vi "test.vi"() -> ()   [LabVIEW 2013]
uses:
  lightfield-automation-labview/LightField Automation.lvclass
panel:
  in  "Delete File?":bool
  in  "Capture Frames":i32=-1
  in  "Capture":bool
  out "Capture ROI 1, Frame 1, Row 2":dbl[](graph)
  out "Acquire ROI 1, Frame 1, Row 1":dbl[](graph)
  in  "Acquire":bool
  in  "ExperimentName":string="Experiment4"
  out "Capture ROI 1, Frame 1":dbl[][](graph)
  out "Acquire ROI 1, Frame 1":dbl[][](graph)
  in  "?":bool
  out "Exposures Per Frame":i32=1
  in  "Exposures Per Frame":i32=1
  out "Number of Frames":i32=1
  in  "Number of Frames":i32=1
  out "Exposure Time (s)":dbl=0.10000000000000009
  in  "Exposure Time (s)":dbl=0.10000000000000009
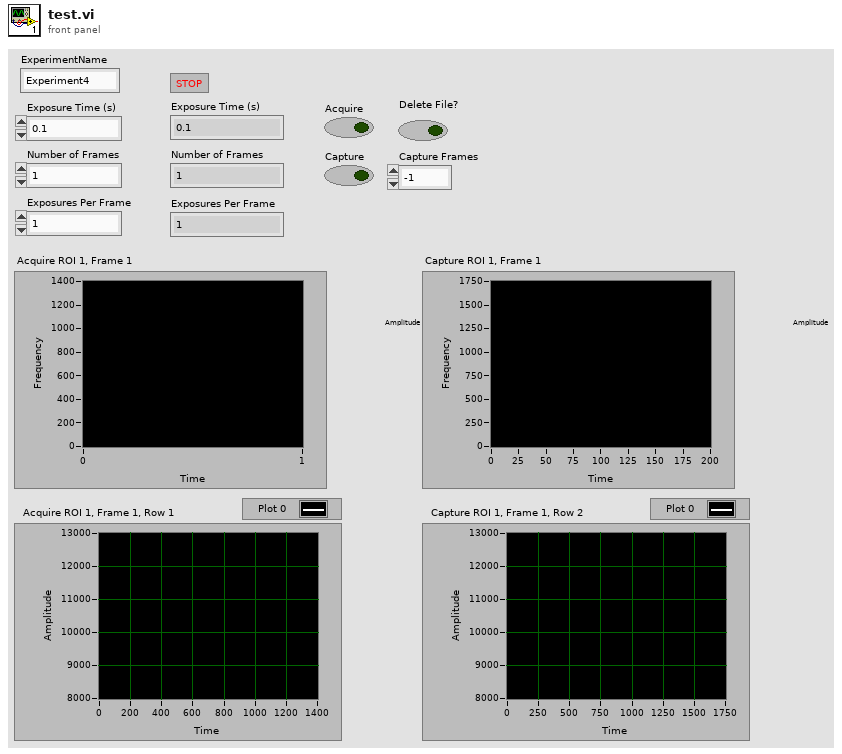
[diagram p1: front panel]
types:
  T1 = cluster{"Image":dbl[][][], "Frame Size":cluster{"F":i32, "Y":i32, "X":i32}}[]
  T2 = cluster{"Image":dbl[][][], "Frame Size":cluster{"F":i32, "Y":i32, "X":i32}}
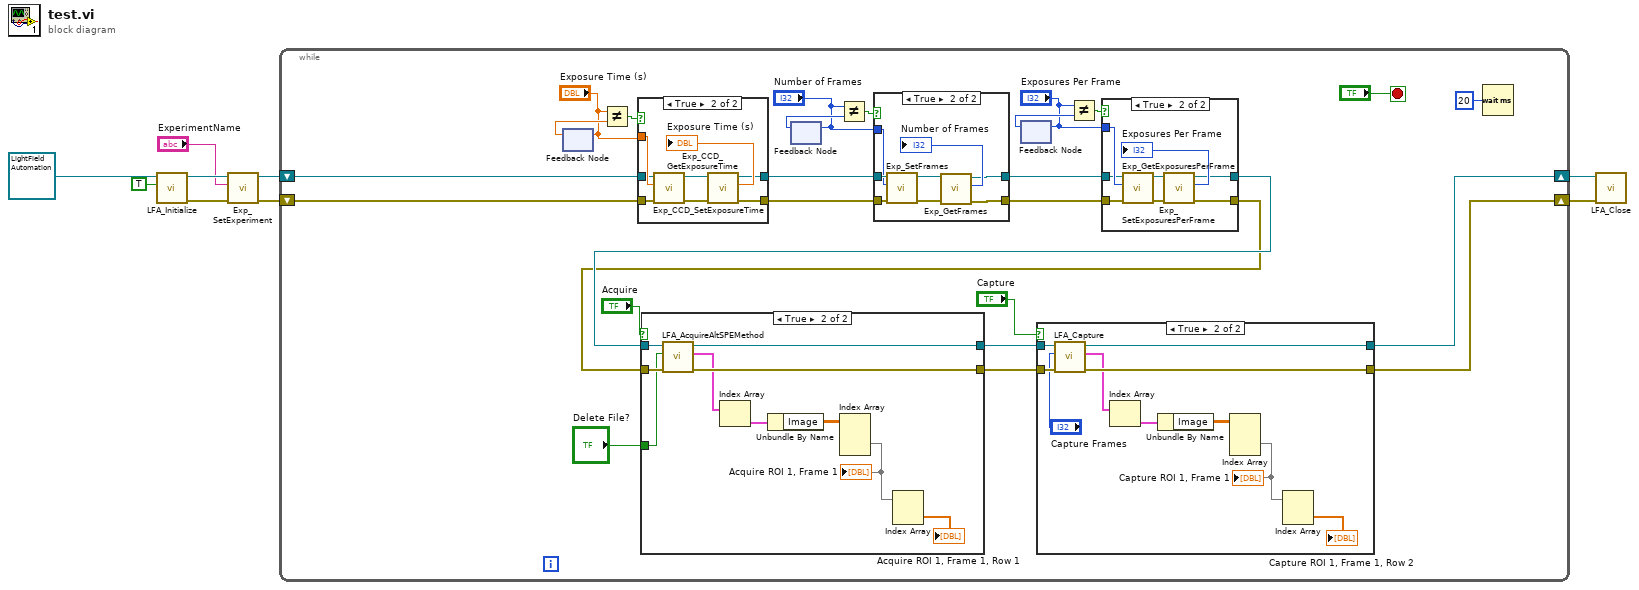
[diagram p0: block diagram]
diagram:
  n1 = call "LFA_Initialize.vi"("Is Visible?"=TRUE, "LightField Automation in"=refnum<class "LightField Automation.lvclass"> refnum ("LightField Automation.lvclass")) -> ("error out"=w6:errorcluster, "LightField Automation out"=w7:refnum<class "LightField Automation.lvclass">)  [unwired: 8 in]
  n2 = call "Exp_SetExperiment.vi"("error in (no error)"=w6, "ExperimentName"="ExperimentName", "LightField Automation in"=w7) -> ("error out"=w5:errorcluster, "LightField Automation out"=w4:refnum<class "LightField Automation.lvclass">)  [unwired: 7 in]
  n3 = while {
    shift-right: [w15] -> w2
    shift-left: w4 -> [w11]
    shift-right: [w14] -> w1
    shift-left: w5 -> [w10]
    stop <- "?" stop-if-true
    n4 = feedback-in #1("Exposure Time (s)") -> ()
    n5 = feedback #1() -> (w32:dbl)  [unwired: 1 in]
    n6 = Not Equal?(x="Exposure Time (s)", y=w32) -> (x != y?=w33:bool)
    n7 = case shown="True" w33 {
      tunnel: "Exposure Time (s)" -> [_ w86]
      tunnel: w11 -> [w80 w85]
      tunnel: w10 -> [w81 w84]
      tunnel: [w80 w83] -> w30
      tunnel: [w81 w82] -> w29
      frame False {
      }
      frame True {
        n8 = call "Exp_CCD_SetExposureTime.vi"("error in (no error)"=w84, "Exposure Time (s)"=w86, "LightField Automation in"=w85) -> ("error out"=w87:errorcluster, "LightField Automation out"=w88:refnum<class "LightField Automation.lvclass">)  [unwired: 7 in]
        n9 = call "Exp_CCD_GetExposureTime.vi"("error in (no error)"=w87, "LightField Automation in"=w88) -> ("error out"=w82:errorcluster, "Exposure Time (s)"=→"Exposure Time (s)":dbl, "LightField Automation out"=w83:refnum<class "LightField Automation.lvclass">)  [unwired: 7 in]
      }
    }
    n10 = feedback #2() -> (w28:i32)  [unwired: 1 in]
    n11 = feedback-in #2("Number of Frames") -> ()
    n12 = Not Equal?(x="Number of Frames", y=w28) -> (x != y?=w27:bool)
    n13 = case shown="True" w27 {
      tunnel: w30 -> [w71 w76]
      tunnel: w29 -> [w70 w75]
      tunnel: "Number of Frames" -> [_ w74]
      tunnel: [w71 w73] -> w22
      tunnel: [w70 w72] -> w21
      frame False {
      }
      frame True {
        n14 = call "Exp_SetFrames.vi"("error in (no error)"=w75, "Number of Frames"=w74, "LightField Automation in"=w76) -> ("error out"=w78:errorcluster, "LightField Automation out"=w79:refnum<class "LightField Automation.lvclass">)  [unwired: 7 in]
        n15 = call "Exp_GetFrames.vi"("error in (no error)"=w78, "LightField Automation in"=w79) -> ("error out"=w72:errorcluster, "Frames"=→"Number of Frames":i32, "LightField Automation out"=w73:refnum<class "LightField Automation.lvclass">)  [unwired: 7 in]
      }
    }
    n16 = feedback #3() -> (w25:i32)  [unwired: 1 in]
    n17 = feedback-in #3("Exposures Per Frame") -> ()
    n18 = Not Equal?(x="Exposures Per Frame", y=w25) -> (x != y?=w24:bool)
    n19 = case shown="True" w24 {
      tunnel: "Exposures Per Frame" -> [_ w66]
      tunnel: w22 -> [w61 w65]
      tunnel: w21 -> [w60 w64]
      tunnel: [w60 w63] -> w18
      tunnel: [w61 w62] -> w20
      frame False {
      }
      frame True {
        n20 = call "Exp_SetExposuresPerFrame.vi"("error in (no error)"=w64, "Exposures Per Frame"=w66, "LightField Automation in"=w65) -> ("error out"=w69:errorcluster, "LightField Automation out"=w68:refnum<class "LightField Automation.lvclass">)  [unwired: 7 in]
        n21 = call "Exp_GetExposuresPerFrame.vi"("error in (no error)"=w69, "LightField Automation in"=w68) -> ("error out"=w63:errorcluster, "Exposures Per Frame"=→"Exposures Per Frame":i32, "LightField Automation out"=w62:refnum<class "LightField Automation.lvclass">)  [unwired: 7 in]
      }
    }
    n22 = case shown="True" "Acquire" {
      tunnel: w20 -> [w49 w55]
      tunnel: w18 -> [w48 w54]
      tunnel: [w49 w52] -> w17
      tunnel: [w48 w51] -> w16
      tunnel: "Delete File?" -> [_ w53]
      frame False {
      }
      frame True {
        n23 = call "LFA_AcquireAltSPEMethod.vi"("error in (no error)"=w54, "Delete File?"=w53, "LightField Automation in"=w55) -> ("error out"=w51:errorcluster, "Data"=w50:T1, "LightField Automation out"=w52:refnum<class "LightField Automation.lvclass">)  [unwired: 6 in]
        n24 = Index Array(array=w50) -> (element=w59:T2)  [unwired: 1 in]
        n25 = Unbundle By Name(w59) -> ("Image"=w58:dbl[][][])
        n26 = Index Array(array=w58) -> (element=w57:dbl[][])  [unwired: 3 in]
        "Acquire ROI 1, Frame 1" <- w57
        n27 = Index Array(array=w57) -> (element=→"Acquire ROI 1, Frame 1, Row 1":dbl[])  [unwired: 2 in]
      }
    }
    n28 = case shown="True" "Capture" {
      tunnel: w17 -> [w37 w43]
      tunnel: w16 -> [w36 w42]
      tunnel: [w37 w40] -> w15
      tunnel: [w36 w41] -> w14
      frame False {
      }
      frame True {
        n29 = call "LFA_Capture.vi"("error in (no error)"=w42, "Frames"="Capture Frames", "LightField Automation in"=w43) -> ("error out"=w41:errorcluster, "Data"=w39:T1, "LightField Automation out"=w40:refnum<class "LightField Automation.lvclass">)  [unwired: 6 in]
        n30 = Index Array(array=w39) -> (element=w47:T2)  [unwired: 1 in]
        n31 = Unbundle By Name(w47) -> ("Image"=w46:dbl[][][])
        n32 = Index Array(array=w46) -> (element=w44:dbl[][])  [unwired: 3 in]
        "Capture ROI 1, Frame 1" <- w44
        n33 = Index Array(array=w44) -> (element=→"Capture ROI 1, Frame 1, Row 2":dbl[])  [unwired: 2 in]
      }
    }
    n34 = Wait (ms)(milliseconds to wait=u32 20) -> ()  [unwired: 1 out]
  }
  n35 = call "LFA_Close.vi"("error in (no error)"=w1, "LightField Automation in"=w2) -> ()  [unwired: 8 in, 2 out]
